vi "Tetra_VmonFullTest.vi"(0 "COMPORT":refnum<visa-resource-name>="COM4", 11 "error in (no error)":errorcluster, 12 "Open Ser(t)":bool, 13 "Clear errors in(t)":bool, 14 "Close Ser(t)":bool) -> (1 "Pass?(T)":bool, 2 "Results":string, 3 "rdv":dbl[](array[numeric]), 4 "comport":refnum<visa-resource-name>="COM4", 15 "error out":errorcluster)   [LabVIEW 2018]
panel:
  in  "new element/subarray":string[](array[string])=["Main Power ", "Vmon(V)", "Vmon_hsl", "Vmon_lsl", "P/F"]
  out "appended array":string[][](array[string])
  in  "y":dbl=0.1 format="%#_13g"
  out "Array":string[](array[string])
  out "V_lsl":dbl[](array[numeric])
  out "V_hsl":dbl[](array[numeric])
  out "Names":string[](array[string])
  out "Rdv":string
  # "Fail Component(refdes), Fail Net Name, Feeds(refdes)[Ux:Uy],Feeds(netname)  Fed By(refdes), Fed By (refdes)"
  # "rdiv\n0)  sw3p6:   186 mA  3600 mV\n1)  sw5p5:    89 mA  5496 mV\n2) sw2p8a:   321 mA  2776 mV\n3) sw2p8b:   334 mA  2768 mV\n4)  sw2p4:  1481 mA  2280 mV\n5)  sw1p4:   556 mA  1360 mV\n>"
  # "0)  isu18p5\n1)  core1p0\n2)   xvr1p0\n3)   dig1p8\n4)   dig3p3\n5)   xvr1p2\n6)   div5p0\n7)   vdd3p3\n8)    rx2p5\n9)    tx2p5"
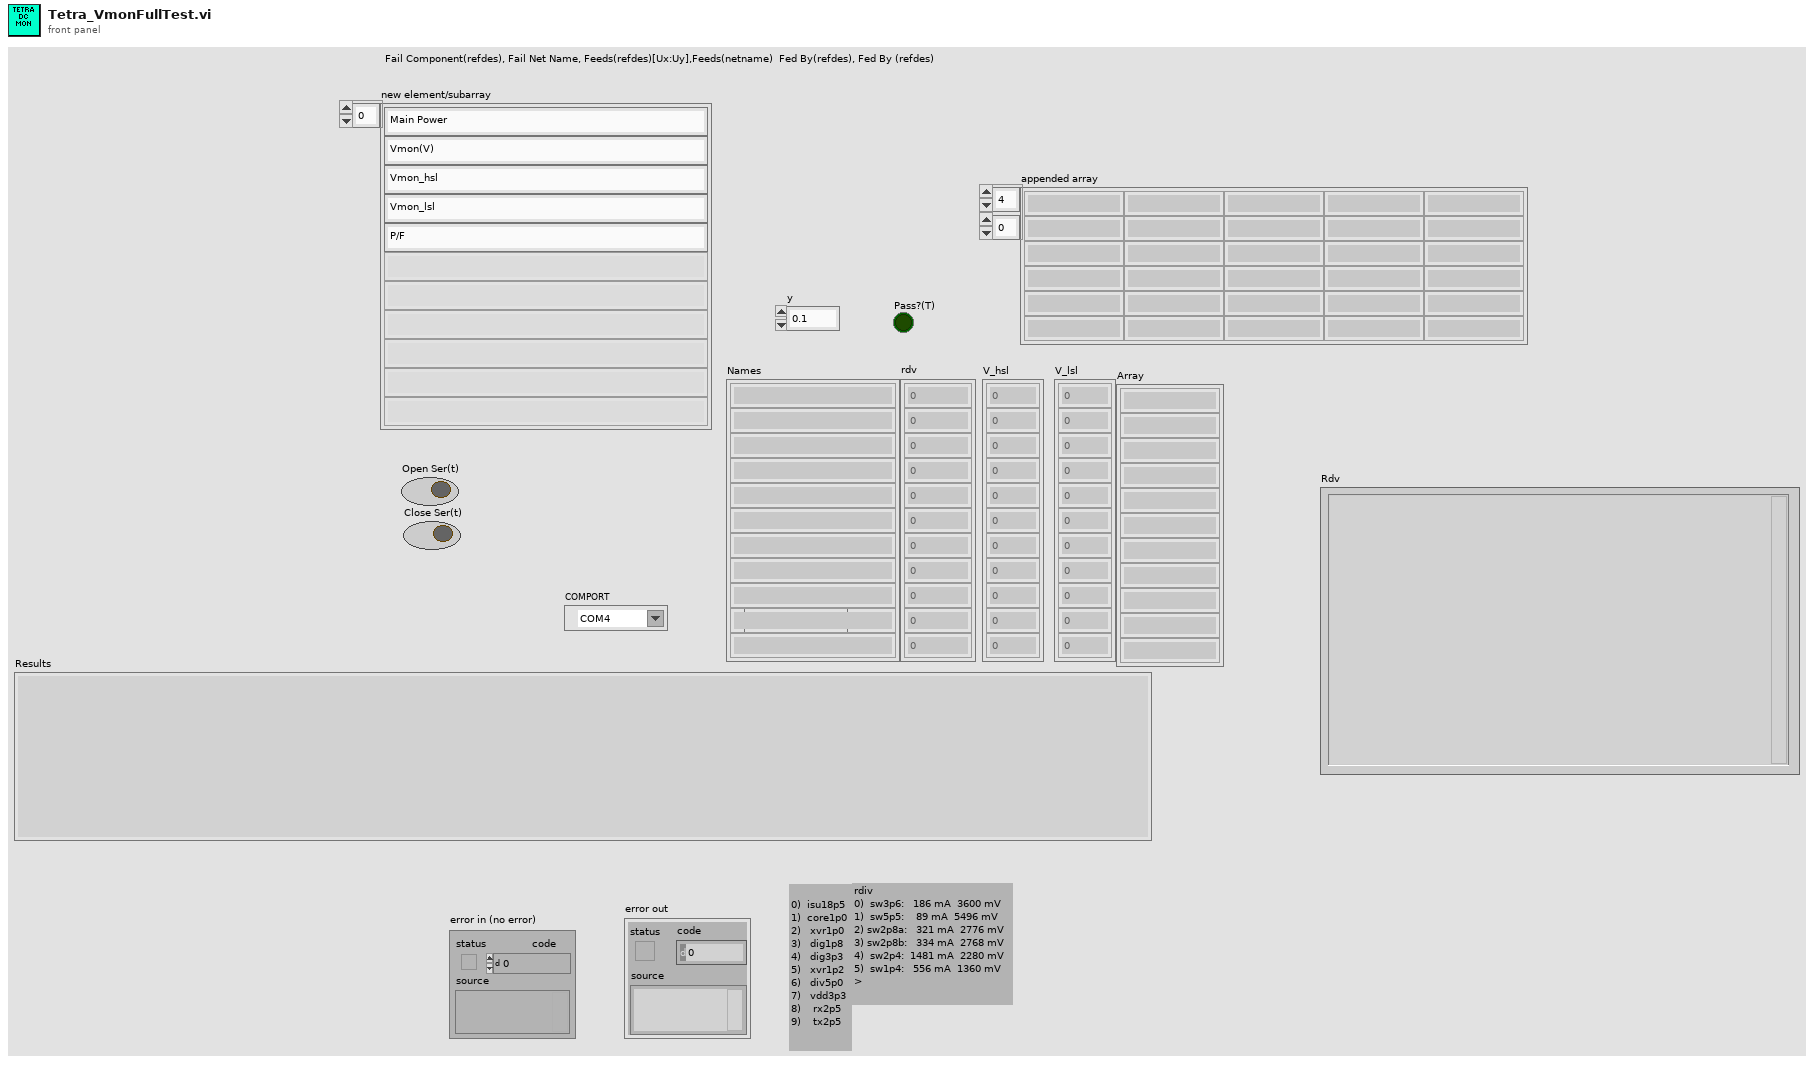
[diagram p1: front panel]
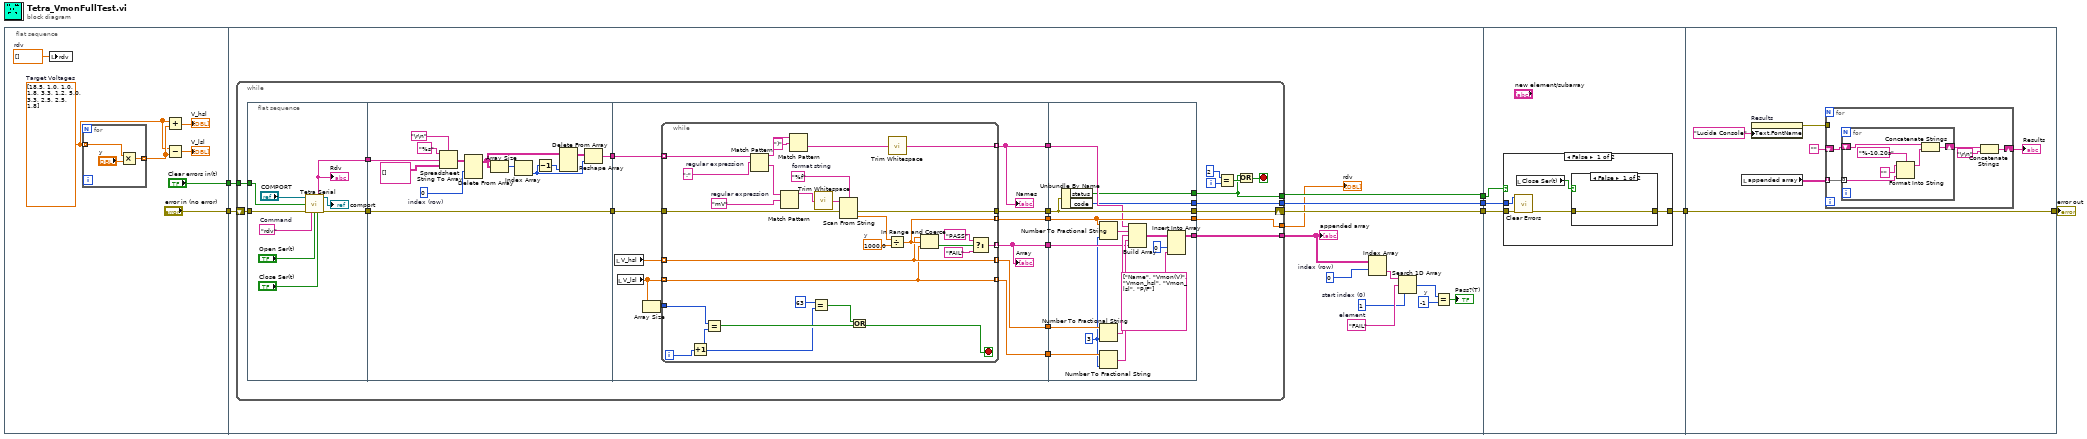
[diagram p0: block diagram]
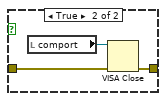
[diagram p2: hidden frame]
diagram:
  n1 = flat-sequence {
    tunnel: ["error in (no error)"] -> w2
    tunnel: ["Clear errors in(t)"] -> w1
    tunnel: [w29] -> w7
    tunnel: [w28] -> w6
    tunnel: [w27] -> w5
    tunnel: w2 -> [w31]
    tunnel: w1 -> [w30]
    tunnel: w7 -> [w133]
    tunnel: w6 -> [w132]
    tunnel: w5 -> [w134]
    tunnel: [w131] -> w3
    tunnel: [w150] -> w4
    tunnel: w3 -> [w150]
    frame #0 {
      w11 = dbl[] [18.5, 1.0, 1.0, 1.8, 3.3, 1.2, 5.0, 3.3, 2.5, 2.5, 1.8]  # Target Voltages
      w10 = dbl[] []  # rdv
      n2 = local write "rdv"(w10) -> ()
      n3 = for {
        tunnel: w11 -> [w17] mode=indexing
        tunnel: [w16] -> w12 mode=indexing
        n4 = Multiply(x=w17, y="y") -> (x*y=w16:dbl)
      }
      n5 = Add(x=w11, y=w12) -> (x+y=→"V_hsl":dbl[])
      n6 = Subtract(x=w11, y=w12) -> (x-y=→"V_lsl":dbl[])
    }
    frame #1 {
      w19 = -1  # y
      w21 = 1  # start index (0)
      w22 = "FAIL"  # element
      w24 = 0  # index (row)
      n7 = while {
        tunnel: w30 -> [w47]
        shift-right: [w35] -> w28
        shift-left: w31 -> [w48]
        tunnel: [w34] -> w29
        tunnel: [w32] -> w27
        tunnel: [w42] -> w26
        tunnel: [w33] -> w25
        i -> [w50]
        stop <- w52 stop-if-true
        n8 = flat-sequence {
          tunnel: w48 -> [w55]
          tunnel: w47 -> [w54]
          tunnel: [w59] -> w46
          tunnel: [w53] -> w45
          tunnel: w46 -> [w74]
          tunnel: w45 -> [w65]
          tunnel: [w74] -> w44
          tunnel: [w62] -> w43
          tunnel: w44 -> [w84]
          tunnel: w43 -> [w85]
          tunnel: [w83] -> w41
          tunnel: [w82] -> w40
          tunnel: [w81] -> w39
          tunnel: [w80] -> w38
          tunnel: [w79] -> w37
          tunnel: [w78] -> w36
          tunnel: [w129] -> w35
          tunnel: [w130] -> w42
          tunnel: w41 -> [w130]
          tunnel: w40 -> [w129]
          tunnel: w39 -> [w125]
          tunnel: w38 -> [w122]
          tunnel: w37 -> [w127]
          tunnel: w36 -> [w128]
          tunnel: [w120] -> w32
          tunnel: [w119] -> w34
          tunnel: [w117] -> w33
          frame #0 {
            w58 = "rdv"  # Command
            n9 = call "Tetra Serial.vi"("COMPORT"="COMPORT", "ClearErrorIn(t)"=w54, "error in (no error)"=w55, "Command"=w58, "Open Ser(t)"="Open Ser(t)", "Close Ser(t)"="Close Ser(t)") -> ("output"=w53:string, "comport"=→"comport":refnum<visa-resource-name>, "error out"=w59:errorcluster)  [unwired: 5 in, 2 out]
            "Rdv" <- w53
          }
          frame #1 {
            w71 = 0  # index (row)
            n10 = Spreadsheet String To Array(delimiter (Tab)="\r\n", format string="%s", spreadsheet string=w65, array type (2D Dbl)=string[][] []) -> (array=w72:string[][])
            n11 = Delete From Array(array=w72, index (row)=w71) -> (array with subset deleted=w66:string[][])  [unwired: 2 in, 1 out]
            n12 = Array Size(array=w66) -> (size(s)=w73:i32[])
            n13 = Index Array(array=w73) -> (element=w67:i32)  [unwired: 1 in]
            n14 = Decrement(x=w67) -> (x-1=w64:i32)
            n15 = Delete From Array(array=w66, index (col)=w64) -> (array with subset deleted=w63:string[][])  [unwired: 2 in, 1 out]
            n16 = Reshape Array(w63, w67) -> (w62:string[])
          }
          frame #2 {
            n17 = local read "V_hsl"() -> (w77:dbl[])
            n18 = local read "V_lsl"() -> (w76:dbl[])
            n19 = Array Size(array=w76) -> (size(s)=w75:i32)
            n20 = while {
              tunnel: w85 -> [w114] mode=indexing
              tunnel: [w99] -> w83 mode=indexing
              tunnel: [w105] -> w82
              tunnel: w84 -> [w104]
              tunnel: [w100] -> w81 mode=indexing
              tunnel: w77 -> [w94] mode=indexing
              tunnel: w76 -> [w93] mode=indexing
              tunnel: [w95] -> w80 mode=indexing
              tunnel: [w94] -> w79 mode=indexing
              tunnel: [w93] -> w78 mode=indexing
              tunnel: w75 -> [w92]
              i -> [w91]
              stop <- w89 stop-if-true
              w106 = "%f"  # format string
              w107 = 1000.0  # y
              w111 = "mV"  # regular expression
              w113 = ":"  # regular expression
              n21 = Increment(x=w91) -> (x+1=w87:i32)
              n22 = Equal?(x=w92, y=w87) -> (x = y?=w90:bool)
              n23 = Match Pattern(string=w114, regular expression=w113) -> (before substring=w103:string, after substring=w112:string)  [unwired: 1 in, 2 out]
              n24 = Match Pattern(string=w112, regular expression=w111) -> (before substring=w110:string)  [unwired: 1 in, 3 out]
              n25 = Match Pattern(string=w103, regular expression=")") -> (after substring=w101:string)  [unwired: 1 in, 3 out]
              n26 = Equal?(x=63, y=w87) -> (x = y?=w88:bool)
              n27 = call <vilib>:"Trim Whitespace.vi"("string"=w110) -> ("trimmed string"=w109:string)  [unwired: 1 in]
              n28 = Scan From String(format string=w106, input string=w109, error in=w104) -> (error out=w105:errorcluster, output 1=w108:dbl)  [unwired: 2 in, 2 out]
              n29 = Or(x=w88, y=w90) -> (x .or. y?=w89:bool)
              n30 = Divide(x=w108, y=w107) -> (x/y=w99:dbl)
              n31 = call <vilib>:"Trim Whitespace.vi"("string"=w101) -> ("trimmed string"=w100:string)  [unwired: 1 in]
              n32 = In Range and Coerce(upper limit=w94, x=w99, lower limit=w93) -> (In Range?=w98:bool)  [unwired: 1 out]
              n33 = Select(t="PASS", s=w98, f="FAIL") -> (s? t:f=w95:string)
            }
            "Array" <- w80
            "Names" <- w81
          }
          frame #3 {
            w121 = i16 3 ("precision (6)")
            n34 = Unbundle By Name(w129) -> ("status"=w120:bool, "code"=w119:i32)
            n35 = Number To Fractional String(number=w130, precision (6)=w121) -> (F-format string=w126:string[])  [unwired: 2 in]
            n36 = Number To Fractional String(number=w127, precision (6)=w121) -> (F-format string=w124:string[])  [unwired: 2 in]
            n37 = Number To Fractional String(number=w128, precision (6)=w121) -> (F-format string=w123:string[])  [unwired: 2 in]
            n38 = Build Array(w125, w126, w124, w123, w122) -> (w118:string[][])
            n39 = Insert Into Array(array=w118, index (col)=0 ("disabled index (col)"), new element=string[] ["Name", "Vmon(V)", "Vmon_hsl", "Vmon_lsl", "P/F"] ("new element/subarray")) -> (w117:string[][])  [unwired: 1 in]
          }
        }
        n40 = Equal?(x=2, y=w50) -> (x = y?=w51:bool)
        n41 = Or(x=w32, y=w51) -> (x .or. y?=w52:bool)
      }
      "rdv" <- w26
      "appended array" <- w25
      n42 = Index Array(array=w25, index (row)=w24) -> (element=w23:string[])  [unwired: 1 in]
      n43 = Search 1D Array(1D array=w23, element=w22, start index (0)=w21) -> (index of element=w20:i32)
      n44 = Equal?(x=w20, y=w19) -> (x = y?=→"Pass?(T)":bool)
    }
    frame #2 {
      n45 = case shown="False" w134 {
        tunnel: w133 -> [w139 _]
        tunnel: w132 -> [w137 w144]
        tunnel: [w136 w144] -> w131
        frame False {
          n46 = call <vilib>:"Clear Errors.vi"("error in (no error)"=w137, "specific error code to clear (0: all)"=w139) -> ("error out"=w138:errorcluster)  [unwired: 4 in, 1 out]
          n47 = local read "Close Ser(t)"() -> (w135:bool)
          n48 = case shown="False" w135 {
            tunnel: w138 -> [w140 w142]
            tunnel: [w140 w141] -> w136
            frame False {
            }
            frame True {
              n49 = local read "comport"() -> (w143:refnum<visa-resource-name>)
              n50 = VISA Close(VISA resource name=w143, error in (no error)=w142) -> (error out=w141:errorcluster)
            }
          }
        }
        frame True {
        }
      }
    }
    frame #3 {
      n51 = local read "appended array"() -> (w145:string[][])
      n52 = property on="Results" class="Str"("Text.FontName"="Lucida Console" ("Text.Font:Name")) -> (error out=w148:errorcluster)  [unwired: 2 in, 1 out]
      n53 = for {
        tunnel: w145 -> [w155] mode=indexing
        shift-right: [w153] -> w149
        shift-left: "" -> [w151]
        tunnel: w148 -> [_]
        n54 = for {
          tunnel: w155 -> [w160] mode=indexing
          shift-right: [w158] -> w154
          shift-left: w151 -> [w156]
          n55 = Format Into String(format string="%-10.20s", initial string="", w160) -> (resulting string=w159:string)  [unwired: 1 in, 1 out]
          n56 = Concatenate Strings(w156, w159) -> (w158:string)
        }
        n57 = Concatenate Strings(w154, "\r\n") -> (w153:string)
      }
      "Results" <- w149
    }
  }
  "error out" <- w4
